vi "Active Project Scope Index.vi"(8 "Error In":errorcluster, 10 "Strings[]":string[](array[string]), 11 "App In":refnum<vi>) -> (0 "Error Out":errorcluster, 2 "Index":i32=-1, 3 "App Out":refnum<vi>)   [LabVIEW 2017, in "Bookmark Manager.lvlib"]
doc: "Determines which project to use for the scope from the list of projects that will be used for the scope's ring."
uses:
  Bookmark Manager.lvlib
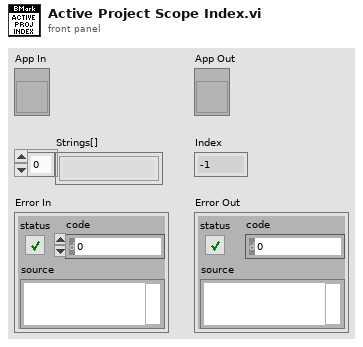
[diagram p1: front panel]
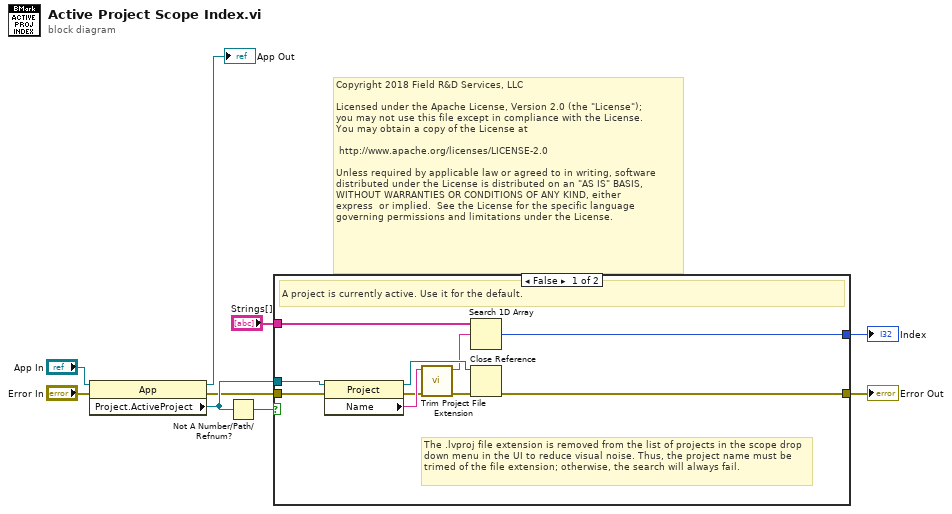
[diagram p0: block diagram]
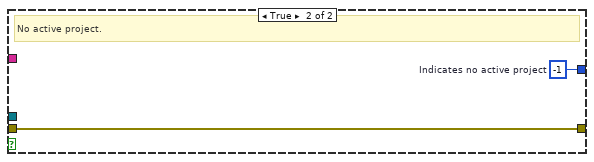
[diagram p2: hidden frame]
diagram:
  # "Copyright 2018 Field R&D Services, LLC\n\nLicensed under the Apache License, Version 2.0 (the \"License\");\nyou may not use this file except in compliance with the License.\nYou may obtain a copy of the License at\n\n\thttp://www.apache.org/licenses/LICENSE-2.0\n\nUnless required by applicable law or agreed to in writing, software\ndistributed under the License is distributed on an \"AS IS\" BASIS,\nWITHOUT WARRANTIES OR CONDITIONS OF ANY KIND, either \nexpress  or implied.  See the License for the specific language \ngoverning permissions and limitations under the License."
  n1 = property class="App"(reference="App In", error in="Error In") -> (reference out=→"App Out":refnum<vi>, error out=w6:errorcluster, "Project.ActiveProject"=w7:refnum<vi>)
  n2 = Not A Number/Path/Refnum?(number/path/refnum=w7) -> (NaN/Path/Refnum?=w5:bool)
  n3 = case shown="False" w5 {
    tunnel: w6 -> [w18 w21]
    tunnel: w7 -> [w19 _]
    tunnel: [w16 w21] -> w8
    tunnel: "Strings[]" -> [w15 _]
    tunnel: [w13 w20] -> w1
    frame False {
      # "The .lvproj file extension is removed from the list of projects in the scope drop down menu in the UI to reduce visual noise. Thus, the project name must be trimed of the file extension; otherwise, the search will always fail."
      # "A project is currently active. Use it for the default."
      n4 = property class="Project"(reference=w19, error in=w18) -> (reference out=w17:refnum<vi>, error out=w11:errorcluster, "Name"=w14:string)
      n5 = call "Trim Project File Extension.vi"("Error In"=w11, "Project File Name"=w14) -> ("Error Out"=w10:errorcluster, "Project Name"=w12:string)  [unwired: 8 in]
      n6 = Search 1D Array(1D array=w15, element=w12) -> (index of element=w13:i32)  [unwired: 1 in]
      n7 = Close Reference(reference=w17, error in (no error)=w10) -> (error out=w16:errorcluster)
    }
    frame True {
      w20 = -1  # Indicates no active project
      # "No active project."
    }
  }
  "Error Out" <- w8
  "Index" <- w1
